vi "Launch GUI.vi"(8 "error in (no error)":errorcluster, 11 "GUI Builder in":refnum<class "GUI Builder.lvclass">) -> (0 "error out":errorcluster)   [LabVIEW 2021, in "App-Builder Library.lvlib" / "GUI Builder.lvclass"]
uses:
  GUI Builder.lvclass
  GUI.vi
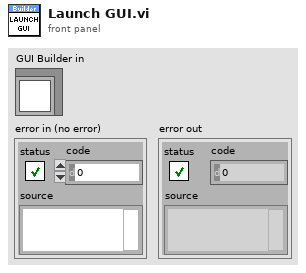
[diagram p1: front panel]
types:
  T1 = enum32{"Bad", "Idle", "Run top level", "Running"}
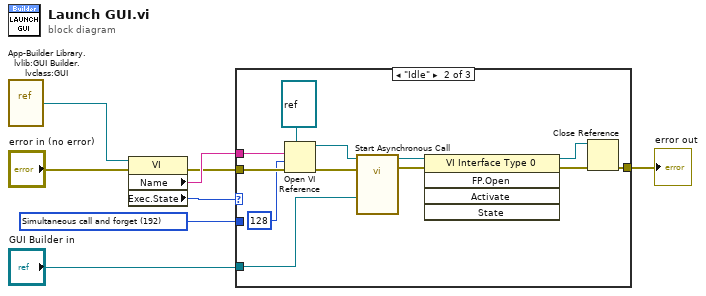
[diagram p0: block diagram]
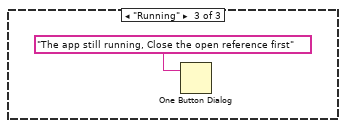
[diagram p3: hidden frame]
diagram:
  w1 = 192 items=["Record modifications"=1, "Open templates for editing"=2, "Prompt user to save"=4, "Prepare for reentrant run"=8, "Prompt to find missing subVIs"=16, "Hide loading dialog box"=32, "Enable simultaneous calls"=64, "Call and Forget"=80, "Prepare to call and forget"=128, "Simultaneous call and forget"=192, "Prepare to call and collect"=256, "Simultaneous call and collect"=320] ("Ring")
  n1 = vi-ref "App-Builder Library.lvlib:GUI Builder.lvclass:GUI.vi"() -> (w8:refnum<vi>)
  n2 = property class="VI"(reference=w8, error in="error in (no error)") -> (error out=w6:errorcluster, "Name"=w7:string, "Exec.State"=w2:T1)  [unwired: 1 out]
  n3 = case shown="\"Idle\"" w2 {
    tunnel: w7 -> [_ w19 _]
    tunnel: w6 -> [_ w18 _]
    tunnel: [_ w15 _] -> w4
    tunnel: "GUI Builder in" -> [_ w14 _]
    tunnel: w1 -> [_ _ _]
    frame Default {
    }
    frame "Idle" {
      n4 = Open VI Reference(type specifier VI Refnum (for type only)=refnum<vi> refnum, vi path=w19, options=128, error in (no error)=w18) -> (vi reference=w20:refnum<vi>, error out=w17:errorcluster)  [unwired: 2 in]
      n5 = call-by-ref "Start Asynchronous Call"(reference=w20, error in=w17, "GUI Builder in"=w14) -> (reference out=w13:refnum<vi>, error out=w10:errorcluster)  [unwired: 11 in]
      n6 = invoke class="VI Interface Type 0" method="FP.Open"(reference=w13, error in=w10) -> (reference out=w11:refnum<vi>, error out=w12:errorcluster)  [unwired: 3 in, 3 out]
      n7 = Close Reference(reference=w11, error in (no error)=w12) -> (error out=w15:errorcluster)
    }
    frame "Running" {
      n8 = One Button Dialog(message="The app still running, Close the open reference first" ("format string")) -> ()  [unwired: 1 in, 1 out]
    }
  }
  "error out" <- w4
